vi "Exercicio 3.vi"() -> ()   [LabVIEW 2019]
uses:
  <vilib>/Utility/file.llb/Write Delimited Spreadsheet (DBL).vi
panel:
  out "appended array":dbl[][](array[numeric])
  in  "R0":dbl
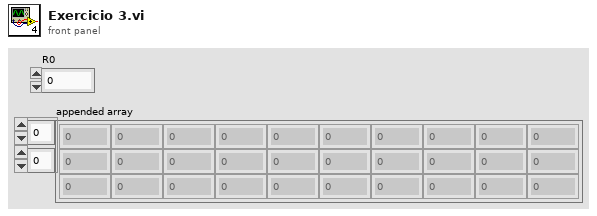
[diagram p1: front panel]
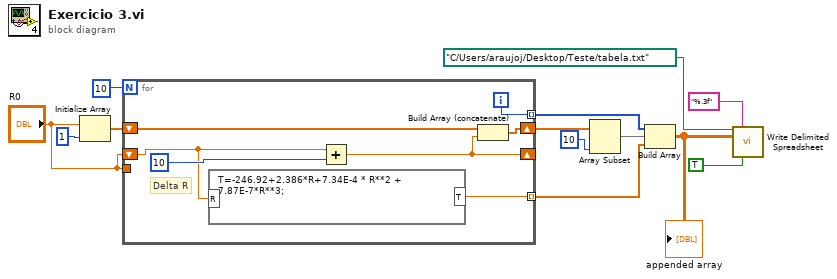
[diagram p0: block diagram]
diagram:
  n1 = Initialize Array("R0", 1) -> (w10:dbl[])
  n2 = for {
    N: 10 -> [_]
    tunnel: "R0" -> [_]
    shift-right: [w15] -> _
    shift-left: "R0" -> [w17]
    tunnel: [w20] -> w3 mode=indexing
    shift-right: [w16] -> w6
    shift-left: w10 -> [w18]
    tunnel: [w14] -> w4 mode=indexing
    i -> [w14]
    # "Delta R"
    n3 = formula code="T=-246.92+2.386*R+7.34E-4 * R**2 + 7.87E-7*R**3;"("R"=w17) -> ("T"=w20:dbl)
    n4 = Add(x=w17, y=10) -> (x+y=w15:dbl)
    n5 = Build Array (concatenate)(w18, w15) -> (w16:dbl[])
  }
  n6 = Array Subset(array=w6, length=10) -> (w2:dbl[])  [unwired: 1 in]
  n7 = Build Array(w4, w2, w3) -> (w1:dbl[][])
  "appended array" <- w1
  n8 = call-poly <vilib>:"Write Delimited Spreadsheet.vi"("file path (dialog if empty)"=path "C:/Users/araujoj/Desktop/Teste/tabela.txt", "format (%.3f)"="%.3f", "2D data"=w1, "transpose? (no:F)"=TRUE) -> ()  [unwired: 10 in, 2 out]
